vi "ExSetEMGain.vi"(2 "error in (no error)":errorcluster, 3 "Readout Port":i32, 4 "EM Gain":i32, 5 "Camera Handle":u32) -> (0 "error out":errorcluster, 1 "Camera Handle Out":u32)   [LabVIEW 2010]
uses:
  Open-Close Hardware/CamHandle.vi
panel:
  # "ExSetEmGain.vi : This vi sets up the \nEM Ggain and EM Gain Port. \nNote: not all cameras support this function."
  # "0 - EM Port\n1 - Normal\n2 - Last"
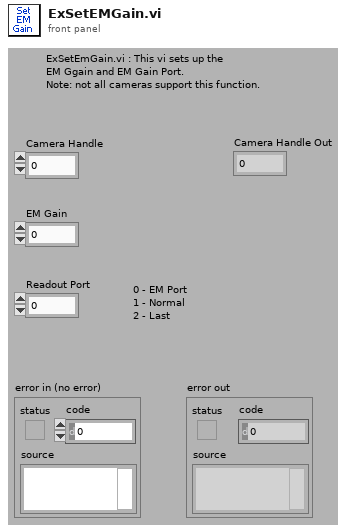
[diagram p1: front panel]
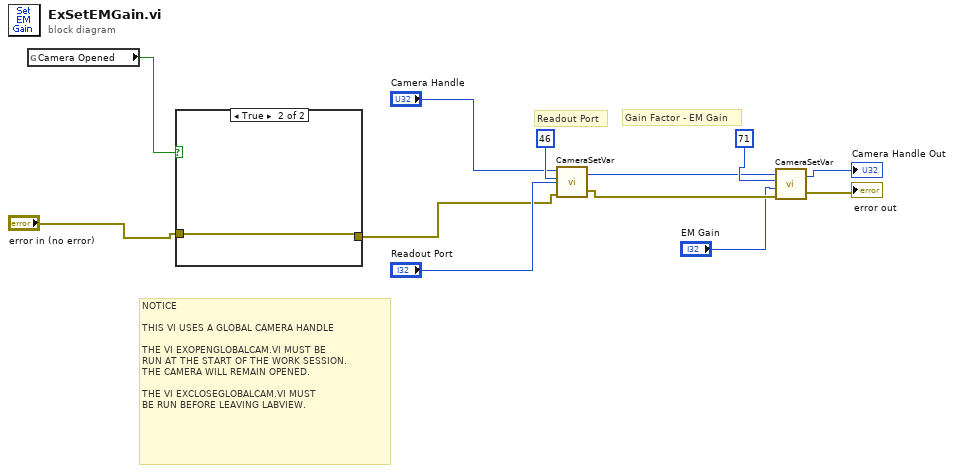
[diagram p0: block diagram]
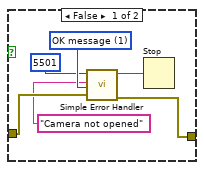
[diagram p2: hidden frame]
diagram:
  # "NOTICE\n\nTHIS VI USES A GLOBAL CAMERA HANDLE\n\nTHE VI EXOPENGLOBALCAM.VI MUST BE\nRUN AT THE START OF THE WORK SESSION.\nTHE CAMERA WILL REMAIN OPENED.\n\nTHE VI EXCLOSEGLOBALCAM.VI MUST\nBE RUN BEFORE LEAVING LABVIEW."
  # "Readout Port"
  # "Gain Factor - EM Gain"
  n1 = global read "CamHandle.vi" "Camera Opened"() -> (w1:bool)
  n2 = case shown="True" w1 {
    tunnel: "error in (no error)" -> [w17 w19]
    tunnel: [w16 w19] -> w2
    frame False {
      w18 = u16 1 items=["no dialog", "OK message", "continue or stop message"] ("type of dialog (OK msg:1)")
      n3 = call <vilib>:"Simple Error Handler.vi"("error code (no error:0)"=5501, "error source (\" \")"="Camera not opened", "type of dialog (OK msg:1)"=w18, "error in (no error)"=w17) -> ("error?"=w14:bool, "error out"=w16:errorcluster)  [unwired: 1 in, 3 out]
      n4 = Stop(stop? (T)=w14) -> ()
    }
    frame True {
    }
  }
  n5 = call <userlib>:"CameraSetVar.vi"("error in"=w2, "Value"="Readout Port", "Parameter ID"=46, "Camera Handle"="Camera Handle") -> ("error out"=w5:errorcluster, "CameraHandle"=w9:u32)
  n6 = call <userlib>:"CameraSetVar.vi"("error in"=w5, "Value"="EM Gain", "Parameter ID"=71, "Camera Handle"=w9) -> ("error out"=→"error out":errorcluster, "CameraHandle"=→"Camera Handle Out":u32)
